vi "Index Prepared Statements.vi"(8 "error in (no error)":errorcluster, 11 "SQLite3LV Connection in":refnum<class "sqlite3.lvclass">) -> (0 "error out":errorcluster, 1 "pStmt":i64[](array[numeric]), 2 "zSQL":string[](array[string]), 3 "SQLite3LV Connection out":refnum<class "sqlite3.lvclass">)   [LabVIEW 2014, in "SQLite3LV.lvlib" / "sqlite3.lvclass"]
uses:
  sqlite3.lvclass
  sqlite3_64.dll
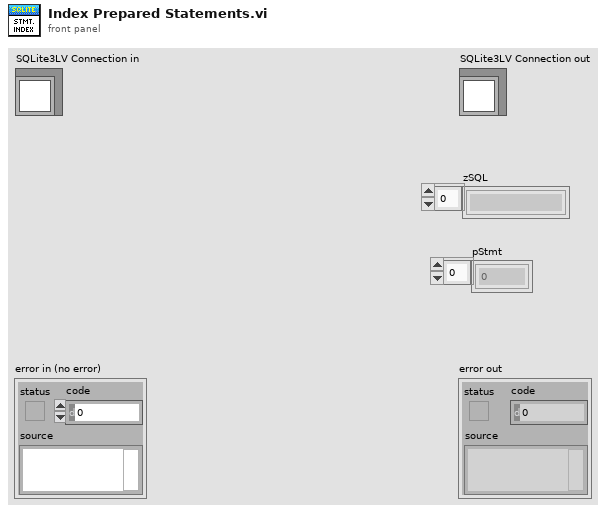
[diagram p1: front panel]
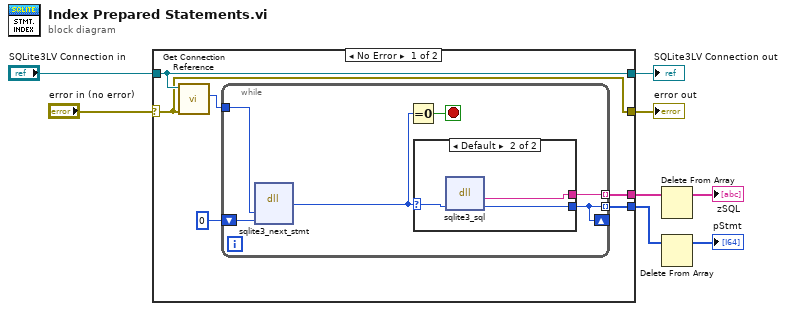
[diagram p0: block diagram]
diagram:
  n1 = case shown="No Error" "error in (no error)" {
    selector: "error in (no error)" -> [w13 w26]
    tunnel: [w13 w26] -> w7
    tunnel: [w14 w25] -> w5
    tunnel: "SQLite3LV Connection in" -> [w14 w25]
    tunnel: [w10 _] -> w4
    tunnel: [w9 _] -> w2
    frame No Error {
      n2 = call "Get Connection Reference.vi"("error in (no error)"=w13, "SQLite3LV Connection in"=w14) -> ("ppDb"=w11:i64)  [unwired: 7 in, 2 out]
      n3 = while {
        shift-right: [w15] -> _
        shift-left: i64 0 ("pStmt") -> [w19]
        tunnel: w11 -> [w20]
        tunnel: [w17] -> w10 mode=indexing
        tunnel: [w15] -> w9 mode=indexing
        stop <- w18 stop-if-true
        n4 = dll-call lib="C:/Users/BobUser/Desktop/LVTables/sqlite3**.*" fn="sqlite3_next_stmt"("ppDb"=w20, "pStmt"=w19) -> ("psqlite3_stmt"=w16:i64)  [unwired: 5 in, 2 out]
        n5 = Equal To 0?(x=w16) -> (x = 0?=w18:bool)
        n6 = case shown="Default" w16 {
          selector: w16 -> [w21 w22]
          tunnel: [_ w24] -> w17
          tunnel: [w21 w23] -> w15
          frame 0 {
          }
          frame Default {
            n7 = dll-call lib="C:/Users/BobUser/Desktop/LVTables/sqlite3**.*" fn="sqlite3_sql"("pStmt"=w22) -> ("zSQL"=w24:string, "pStmt"=w23:i64)  [unwired: 3 in, 2 out]
          }
        }
      }
    }
    frame Error {
    }
  }
  "error out" <- w7
  "SQLite3LV Connection out" <- w5
  n8 = Delete From Array(array=w4) -> (array with subset deleted=→"zSQL":string[])  [unwired: 2 in, 1 out]
  n9 = Delete From Array(array=w2) -> (array with subset deleted=→"pStmt":i64[])  [unwired: 2 in, 1 out]
